vi "CalculateMotorValues.vi"(0 "Axes":dbl[](array[numeric])) -> (1 "LeftSideMotors":dbl, 2 "RightSideMotors":dbl)   [LabVIEW 2015]
uses:
  Utilities/ShiftGlobals.vi
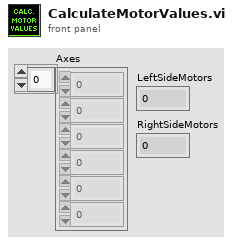
[diagram p1: front panel]
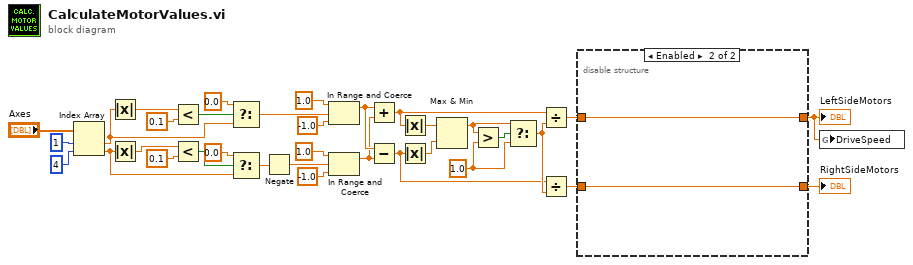
[diagram p0: block diagram]
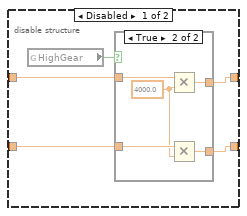
[diagram p2: hidden frame]
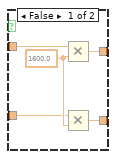
[diagram p3: hidden frame]
diagram:
  w28 = 1.0 ("y")
  n1 = Index Array(array="Axes", index #1=1 ("index"), index #2=4 ("index")) -> (element #1=w4:dbl, element #2=w11:dbl)
  n2 = Absolute Value(x=w4) -> (abs(x)=w6:dbl)
  n3 = Absolute Value(x=w11) -> (abs(x)=w10:dbl)
  n4 = Less?(x=w6, y=0.1) -> (x < y?=w3:bool)
  n5 = Less?(x=w10, y=0.1) -> (x < y?=w8:bool)
  n6 = Select(t=0.0, s=w3, f=w4) -> (s? t:f=w13:dbl)
  n7 = Select(t=0.0, s=w8, f=w11) -> (s? t:f=w12:dbl)
  n8 = Negate(x=w12) -> (-x=w18:dbl)
  n9 = In Range and Coerce(upper limit=1.0, x=w13, lower limit=-1.0) -> (coerced(x)=w20:dbl)  [unwired: 1 out]
  n10 = In Range and Coerce(upper limit=1.0, x=w18, lower limit=-1.0) -> (coerced(x)=w19:dbl)  [unwired: 1 out]
  n11 = Add(x=w20, y=w19) -> (x+y=w26:dbl)
  n12 = Subtract(x=w20, y=w19) -> (x-y=w25:dbl)
  n13 = Absolute Value(x=w26) -> (abs(x)=w32:dbl)
  n14 = Absolute Value(x=w25) -> (abs(x)=w31:dbl)
  n15 = Max & Min(x=w32, y=w31) -> (max(x,y)=w29:dbl)  [unwired: 1 out]
  n16 = Greater?(x=w29, y=w28) -> (0:w30:bool)
  n17 = Select(t=w29, s=w30, f=w28) -> (s? t:f=w27:dbl)
  n18 = Divide(x=w26, y=w27) -> (x/y=w16:dbl)
  n19 = Divide(x=w25, y=w27) -> (x/y=w15:dbl)
  n20 = disable-structure shown="Enabled" {
    disable-tunnel: w16 -> [w39 w51]
    disable-tunnel: w15 -> [w38 w50]
    disable-tunnel: [w36 w50] -> w14
    disable-tunnel: [w35 w51] -> w1
    frame Disabled {
      n21 = global read "ShiftGlobals.vi" "HighGear"() -> (w37:bool)
      n22 = case shown="True" w37 {
        tunnel: w39 -> [w43 w49]
        tunnel: w38 -> [w42 w48]
        tunnel: [w41 w46] -> w35
        tunnel: [w40 w45] -> w36
        frame False {
          w44 = 1600.0 ("y")
          n23 = Multiply(x=w43, y=w44) -> (x*y=w41:dbl)
          n24 = Multiply(x=w42, y=w44) -> (x*y=w40:dbl)
        }
        frame True {
          w47 = 4000.0 ("y")
          n25 = Multiply(x=w49, y=w47) -> (x*y=w46:dbl)
          n26 = Multiply(x=w48, y=w47) -> (x*y=w45:dbl)
        }
      }
    }
    frame Enabled {
    }
  }
  "LeftSideMotors" <- w1
  "RightSideMotors" <- w14
  n27 = global write "ShiftGlobals.vi" "DriveSpeed"(w1) -> ()
